vi "UpdateUIForSelectedDevice.vi"(8 "error in":errorcluster, 9 "Controller Name":string, 10 "UI":T1) -> (0 "error out":errorcluster)   [LabVIEW 2009]
uses:
  Global Variables.vi
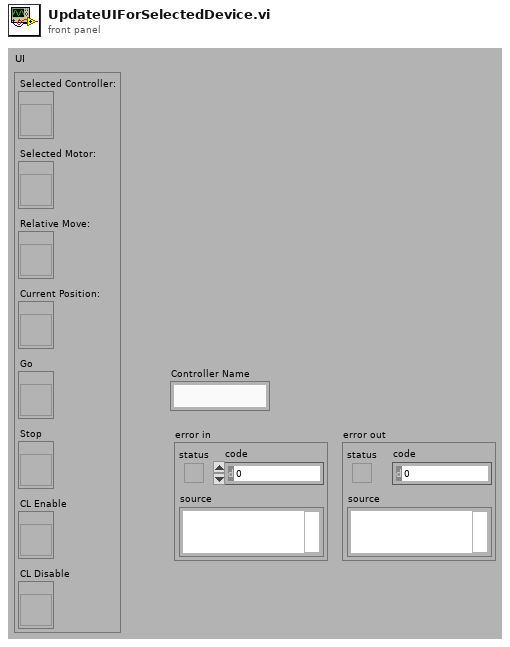
[diagram p1: front panel]
types:
  T1 = cluster{"Selected Controller:":refnum<vi>, "Selected Motor:":refnum<vi>, "Relative Move:":refnum<vi>, "Current Position:":refnum<vi>, "Go":refnum<vi>, "Stop":refnum<vi>, "CL Enable":refnum<vi>, "CL Disable":refnum<vi>}
  T2 = enum8{"Enabled", "Disabled", "Disabled and Grayed Out"}
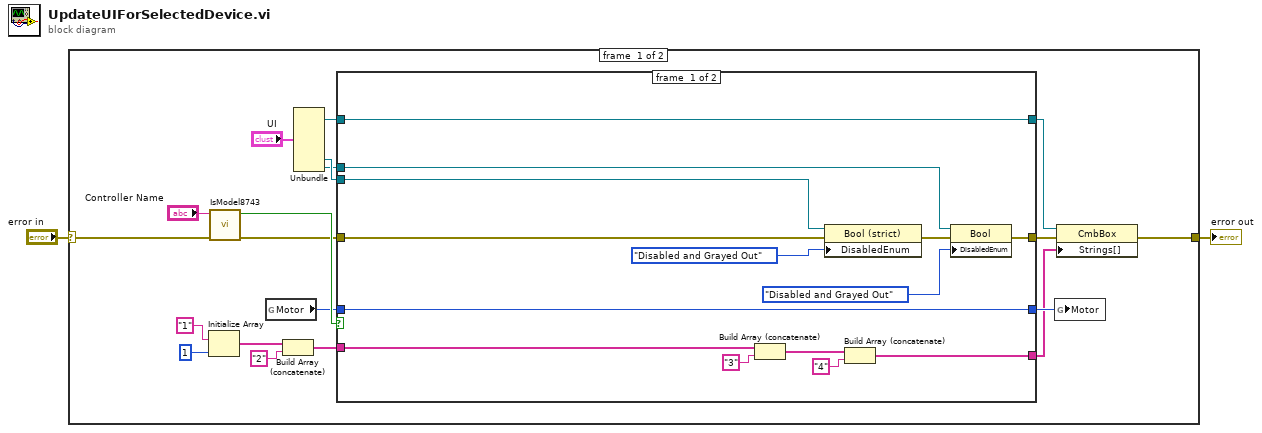
[diagram p0: block diagram]
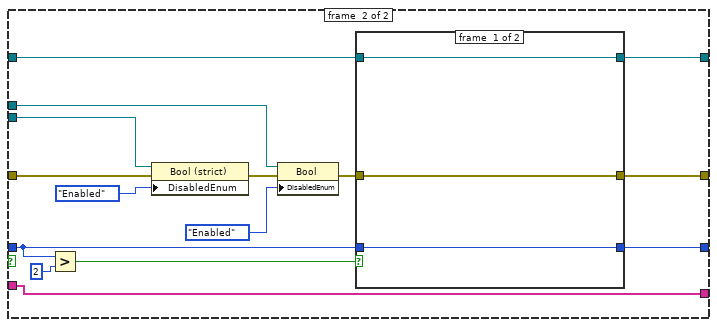
[diagram p2: hidden frame]
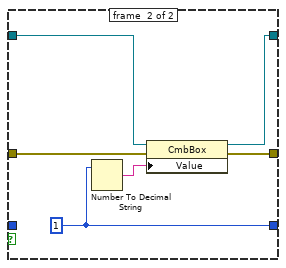
[diagram p3: hidden frame]
diagram:
  n1 = case shown="No Error" "error in" {
    selector: "error in" -> [w8 w60]
    tunnel: [w21 w60] -> w2
    frame #0 {
      n2 = Initialize Array("1", 1 ("dimension size")) -> (w11:string[])
      n3 = call "IsModel8743.vi"("error in"=w8, "Model / Serial"="Controller Name") -> ("error out"=w9:errorcluster, "Boolean"=w10:bool)  [unwired: 8 in]
      n4 = global read "Global Variables.vi" "Motor"() -> (w7:i32)
      n5 = Build Array (concatenate)(w11, "2") -> (w12:string[])
      n6 = Unbundle("UI") -> ("Selected Motor:"=w6:refnum<vi>, "CL Enable"=w5:refnum<vi>, "CL Disable"=w3:refnum<vi>)  [unwired: 5 out]
      n7 = case shown="True" w10 {
        tunnel: w5 -> [w25 w50]
        tunnel: [w34 w45] -> w14
        tunnel: w9 -> [w23 w40]
        tunnel: w7 -> [w33 w43]
        tunnel: w6 -> [w30 w46]
        tunnel: [w33 w44] -> w20
        tunnel: w12 -> [w32 w41]
        tunnel: [w30 w42] -> w13
        tunnel: [w27 w41] -> w18
        tunnel: w3 -> [w24 w38]
        frame #0 {
          n8 = Build Array (concatenate)(w32, "3") -> (w31:string[])
          n9 = property class="Bool (strict)"(reference=w25, error in=w23, "DisabledEnum"=T2."Disabled and Grayed Out" ("Disabled")) -> (error out=w22:errorcluster)  [unwired: 1 out]
          n10 = Build Array (concatenate)(w31, "4") -> (w27:string[])
          n11 = property class="Bool"(reference=w24, error in=w22, "DisabledEnum"=T2."Disabled and Grayed Out" ("Disabled")) -> (error out=w34:errorcluster)  [unwired: 1 out]
        }
        frame #1 {
          n12 = Greater?(x=w43, y=2) -> (0:w47:bool)
          n13 = property class="Bool (strict)"(reference=w50, error in=w40, "DisabledEnum"=T2."Enabled" ("Disabled")) -> (error out=w37:errorcluster)  [unwired: 1 out]
          n14 = property class="Bool"(reference=w38, error in=w37, "DisabledEnum"=T2."Enabled" ("Disabled")) -> (error out=w36:errorcluster)  [unwired: 1 out]
          n15 = case shown="True" w47 {
            tunnel: w46 -> [w51 w58]
            tunnel: w36 -> [w53 w57]
            tunnel: [w53 w55] -> w45
            tunnel: [w52 w59] -> w44
            tunnel: w43 -> [w52 _]
            tunnel: [w51 w54] -> w42
            frame #0 {
            }
            frame #1 {
              w59 = 1 ("number")
              n16 = Number To Decimal String(number=w59) -> (decimal integer string=w56:string)  [unwired: 1 in]
              n17 = property class="CmbBox"(reference=w58, error in=w57, "Value"=w56) -> (reference out=w54:refnum<vi>, error out=w55:errorcluster)
            }
          }
        }
      }
      n18 = global write "Global Variables.vi" "Motor"(w20) -> ()
      n19 = property class="CmbBox"(reference=w13, error in=w14, "Strings[]"=w18) -> (error out=w21:errorcluster)  [unwired: 1 out]
    }
    frame #1 {
    }
  }
  "error out" <- w2
